vi "XY Go.vi"(6 "return immediately":bool, 8 "error in (no error)":errorcluster, 9 "Speed":dbl, 10 "XY In":dbl[](array[numeric]), 11 "Gantry":refnum<k24>) -> (0 "error out":errorcluster, 2 "XY Out 2":dbl[](array[numeric]), 3 "Gantry  2":refnum<k24>)   [LabVIEW 2020, in "Motion.lvclass"]
uses:
  Motion.lvclass
  C:/Program Files (x86)/Aerotech/A3200/LabVIEW/2010/Bin/Aerotech.A3200.dll
  Program Files (x86)/Aerotech/A3200/LabVIEW/2010/Bin/Aerotech.A3200.dll
  Aerotech.lvlib
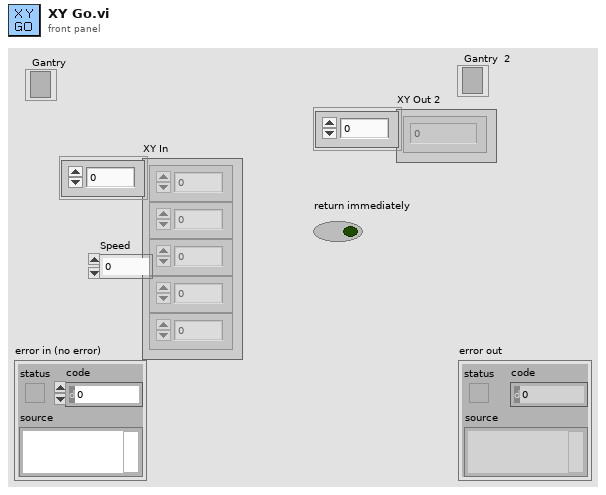
[diagram p1: front panel]
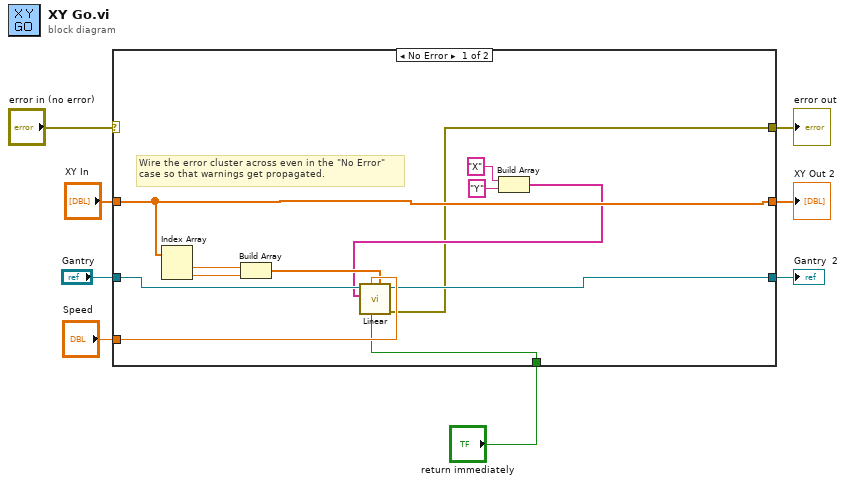
[diagram p0: block diagram]
diagram:
  n1 = case shown="No Error" "error in (no error)" {
    selector: "error in (no error)" -> [_ w23]
    tunnel: [w9 w23] -> w7
    tunnel: "Gantry" -> [w15 w22]
    tunnel: "XY In" -> [w16 w21]
    tunnel: "Speed" -> [w14 _]
    tunnel: [w10 w22] -> w3
    tunnel: [w16 w21] -> w2
    tunnel: "return immediately" -> [w11 _]
    frame No Error {
      # "Wire the error cluster across even in the \"No Error\"\ncase so that warnings get propagated."
      n2 = Index Array(array=w16) -> (element #1=w18:dbl, element #2=w17:dbl)  [unwired: 2 in]
      n3 = Build Array(w18, w17) -> (w13:dbl[])
      n4 = Build Array("X" ("format string"), "Y" ("format string")) -> (w12:string[])
      n5 = call "Linear.vi"("distances"=w13, "return immediately"=w11, "speed"=w14, "axis names"=w12, "controller in"=w15) -> ("error out"=w9:errorcluster, "controller out"=w10:refnum<k24>)  [unwired: 5 in]
    }
    frame Error {
    }
  }
  "error out" <- w7
  "Gantry  2" <- w3
  "XY Out 2" <- w2
